vi "Discard Pic Get Frame.vi"(8 "error in (no error)":errorcluster, 9 "frames":T2, 10 "Img Data indexed":cluster{"image data":T1, "bitmap":u32[][]}, 11 "LF2R IDE in":refnum<class "Main Panel.lvclass">) -> (0 "error out":errorcluster, 3 "LF2R IDE out":refnum<class "Main Panel.lvclass">)   [LabVIEW 2018]
uses:
  Picture Process/Picture Process.lvclass
  <vilib>/picture/picture.llb/Draw True-Color Pixmap.vi
  Main Panel.lvclass
  D:/project/hobby/LabVIEW/LF2R/LabVIEW/Source/Actor/Framework/Framework/Framework.lvclass
  C:/Program Files (x86)/National Instruments/LabVIEW 2018/vi.lib/MGI/Panel Manager/Panel Actor/Panel Actor/Panel Actor.lvclass
  C:/Program Files (x86)/National Instruments/LabVIEW 2018/vi.lib/MGI/Monitored Actor/Monitored Actor/Monitored Actor/Monitored Actor.lvclass
  C:/Program Files (x86)/National Instruments/LabVIEW 2018/vi.lib/ActorFramework/Actor/Actor.lvclass
  Image Json Parser/Img Json Frames.ctl
  Image Json Parser/Image Json Parser.lvclass
  <vilib>/picture/picture.llb/imagedata.ctl
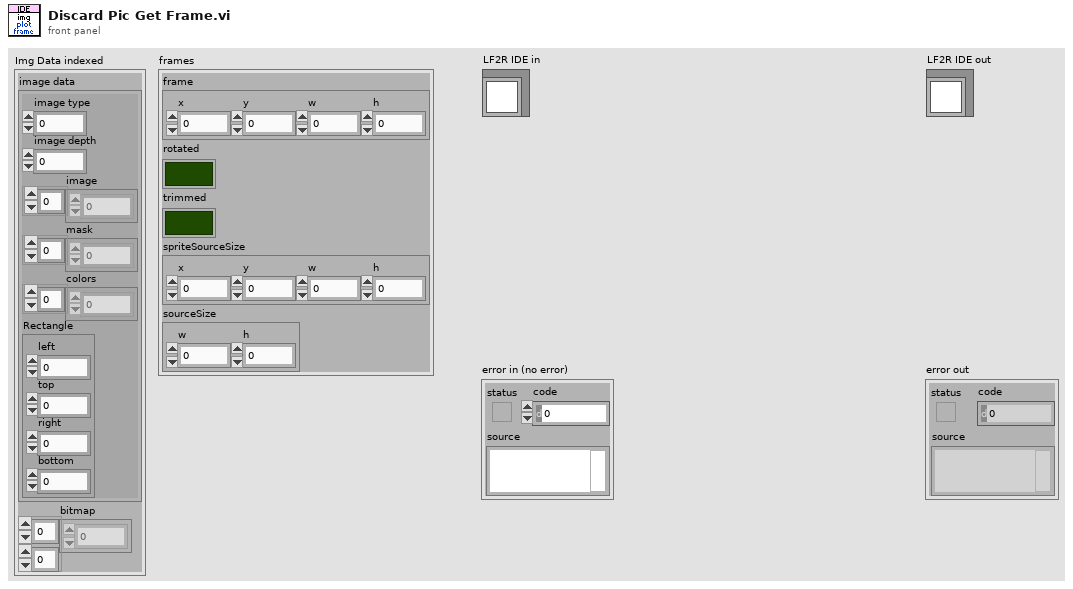
[diagram p1: front panel]
types:
  T1 = typedef "imagedata.ctl" = cluster{"image type":i32, "image depth":i32, "image":u8[], "mask":u8[], "colors":u32[], "Rectangle":cluster{"left":i16, "top":i16, "right":i16, "bottom":i16}}
  T2 = typedef "Image Json Parser.lvclass/Img Json Frames.ctl" = cluster{"frame":cluster{"x":i32, "y":i32, "w":i32, "h":i32}, "rotated":bool, "trimmed":bool, "spriteSourceSize":cluster{"x":i32, "y":i32, "w":i32, "h":i32}, "sourceSize":cluster{"w":i32, "h":i32}}
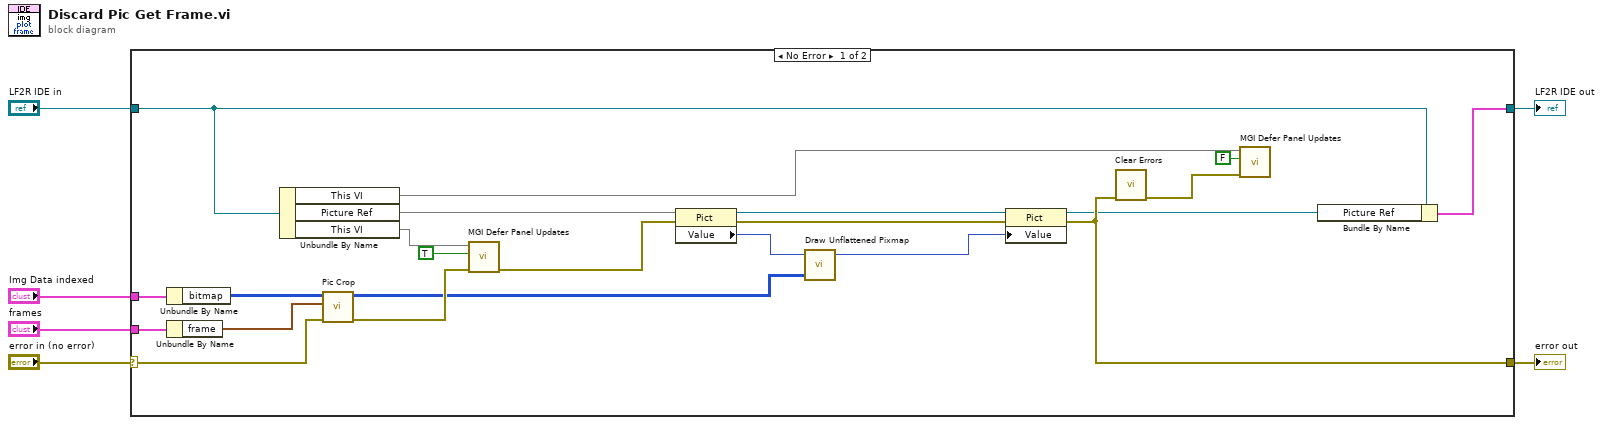
[diagram p0: block diagram]
diagram:
  n1 = case shown="No Error" "error in (no error)" {
    selector: "error in (no error)" -> [w24 w30]
    tunnel: [w10 w30] -> w5
    tunnel: [w7 w29] -> w3
    tunnel: "LF2R IDE in" -> [w9 w29]
    tunnel: "Img Data indexed" -> [w28 _]
    tunnel: "frames" -> [w27 _]
    frame No Error {
      n2 = Unbundle By Name(w28) -> ("bitmap"=w26:u32[][])
      n3 = Unbundle By Name(w27) -> ("frame"=w25:cluster{"x":i32, "y":i32, "w":i32, "h":i32})
      n4 = Unbundle By Name(w9) -> ("This VI"=w11, "Picture Ref"=w16, "This VI"=w22)
      n5 = call "Pic Crop.vi"("error in (no error)"=w24, "Position"=w25, "24-bit pixmap in"=w26) -> ("error out"=w21:errorcluster, "24-bit pixmap out"=w14:u32[][])  [unwired: 7 in]
      n6 = call <userlib>:"MGI Defer Panel Updates.vi"("Error In"=w21, "Defer Updates?"=TRUE, "VI Reference (Caller)"=w22) -> ("Error Out"=w15:errorcluster)  [unwired: 8 in]
      n7 = property class="Pict"(reference=w16, error in=w15) -> (reference out=w19:refnum<vi>, error out=w18:errorcluster, "Value"=w20:picture)
      n8 = call-poly <vilib>:"Draw Unflattened Pixmap.vi"("picture"=w20, "data (RGB format)"=w14) -> ("new picture"=w17:picture)  [unwired: 7 in]
      n9 = property class="Pict"(reference=w19, error in=w18, "Value"=w17) -> (reference out=w8:refnum<vi>, error out=w10:errorcluster)
      n10 = call <vilib>:"Clear Errors.vi"("error in (no error)"=w10) -> ("error out"=w13:errorcluster)  [unwired: 5 in, 1 out]
      n11 = call <userlib>:"MGI Defer Panel Updates.vi"("Error In"=w13, "Defer Updates?"=FALSE, "VI Reference (Caller)"=w11) -> ()  [unwired: 8 in, 1 out]
      n12 = Bundle By Name(cluster=w9, "Picture Ref"=w8) -> (w7:cluster{})
    }
    frame Error {
    }
  }
  "error out" <- w5
  "LF2R IDE out" <- w3
